vi "PH_Interaction.read Database.vi"(3 "error in (no error)":errorcluster, 4 "Strings to search for":string[](array[string]), 5 "DB Entry to read":string) -> (0 "error out":errorcluster, 2 "Values":string[](array[string]))   [LabVIEW 2014, in "PH_Common.lvlib"]
uses:
  PH_Common.lvlib
  CSCore/CSSystem/CSSystemLib/CSSystemLib.lvlib
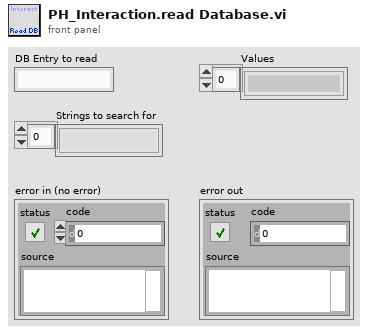
[diagram p1: front panel]
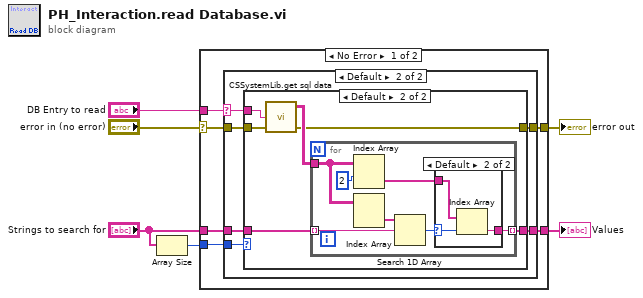
[diagram p0: block diagram]
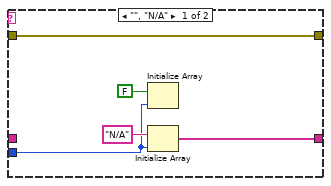
[diagram p2: hidden frame]
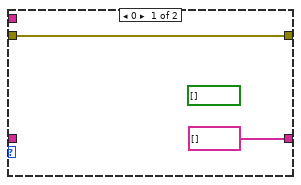
[diagram p3: hidden frame]
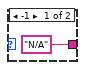
[diagram p4: hidden frame]
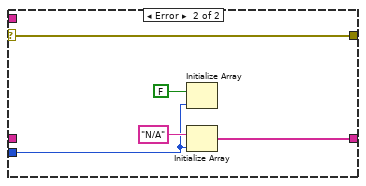
[diagram p5: hidden frame]
diagram:
  n1 = Array Size(array="Strings to search for") -> (size(s)=w1:i32)
  n2 = case shown="No Error" "error in (no error)" {
    selector: "error in (no error)" -> [w9 w47]
    tunnel: [w12 w46] -> w6
    tunnel: "Strings to search for" -> [w11 _]
    tunnel: "DB Entry to read" -> [w8 _]
    tunnel: [w10 w47] -> w4
    tunnel: w1 -> [w7 w43]
    frame No Error {
      n3 = case shown="Default" w8 {
        selector: w8 -> [_ w19]
        tunnel: [w15 w23] -> w12
        tunnel: w11 -> [_ w22]
        tunnel: [w17 w21] -> w10
        tunnel: w9 -> [w17 w20]
        tunnel: w7 -> [w13 w18]
        frame "", "N/A" {
          n4 = Initialize Array(FALSE, w13) -> ()  [unwired: 1 out]
          n5 = Initialize Array("N/A", w13) -> (w15:string[])
        }
        frame Default {
          n6 = case shown="Default" w18 {
            tunnel: [string[] [] w31] -> w23
            tunnel: w22 -> [_ w30]
            tunnel: [w25 w28] -> w21
            tunnel: w20 -> [w25 w27]
            tunnel: w19 -> [_ w26]
            frame 0 {
              (unwired) bool[] []
            }
            frame Default {
              n7 = call "CSSystemLib.get sql data.vi"("error in (no error)"=w27, "object"=w26) -> ("error out"=w28:errorcluster, "queryResults"=w29:string[][])  [unwired: 1 in, 1 out]
              n8 = for {
                tunnel: w30 -> [w36] mode=indexing
                tunnel: w29 -> [w35]
                tunnel: [w32] -> w31 mode=indexing
                n9 = Index Array(array=w35, index (row)=2) -> (element=w34:string[])  [unwired: 1 in]
                n10 = Index Array(array=w35) -> (element=w37:string[])  [unwired: 2 in]
                n11 = Search 1D Array(1D array=w37, element=w36) -> (index of element=w33:i32)  [unwired: 1 in]
                n12 = case shown="Default" w33 {
                  selector: w33 -> [_ w40]
                  tunnel: ["N/A" w42] -> w32
                  tunnel: w34 -> [_ w41]
                  frame -1 {
                  }
                  frame Default {
                    n13 = Index Array(array=w41, index=w40) -> (element=w42:string)
                  }
                }
              }
            }
          }
        }
      }
    }
    frame Error {
      n14 = Initialize Array(FALSE, w43) -> ()  [unwired: 1 out]
      n15 = Initialize Array("N/A", w43) -> (w46:string[])
    }
  }
  "Values" <- w6
  "error out" <- w4
